vi "Decompose VI (Path).vi"(8 "Error in":errorcluster caption="Error in (no error)", 11 "VI path":path) -> (0 "Error out":errorcluster, 1 "Block Diagram XML":string, 2 "Front Panel XML":string, 3 "VI path out":path, 4 "Other resources":T1)   [LabVIEW 2023]
uses:
  CTLs/Resource Array.ctl
  CTLs/Resource.ctl
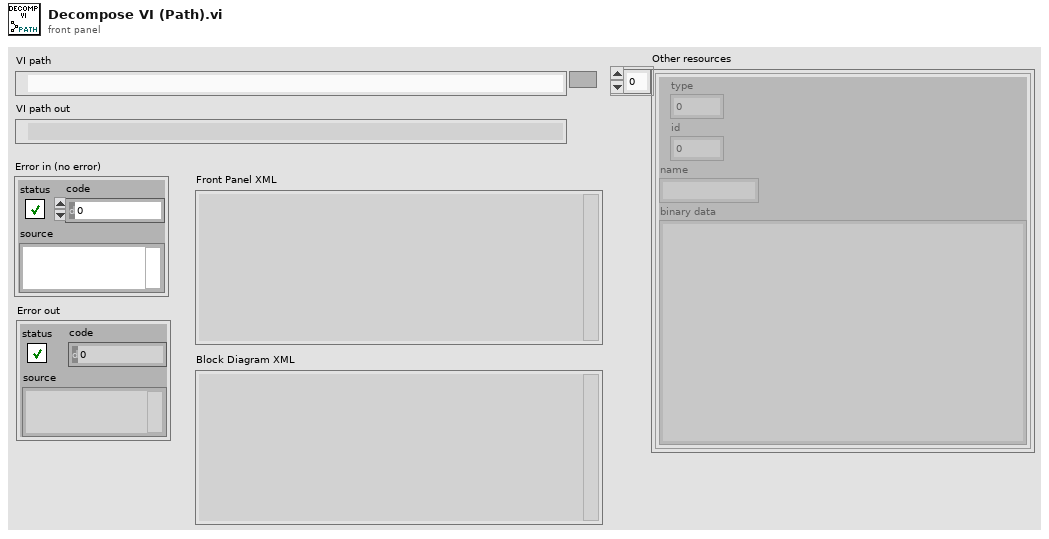
[diagram p1: front panel]
types:
  T1 = typedef "Resource Array.ctl" = T2[]
  T2 = typedef "Resource.ctl" = cluster{"type":u32, "id":i32, "name":string, "binary data":string}
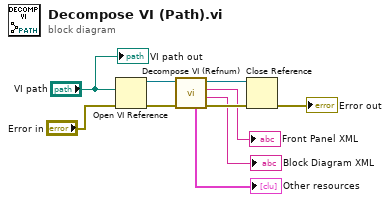
[diagram p0: block diagram]
diagram:
  n1 = Open VI Reference(vi path="VI path", error in (no error)="Error in") -> (vi reference=w10:refnum<vi>, error out=w9:errorcluster)  [unwired: 4 in]
  n2 = call "Decompose VI (Refnum).vi"("Error in"=w9, "VI Refnum"=w10) -> ("Error out"=w6:errorcluster, "Block Diagram XML"=→"Block Diagram XML":string, "Front Panel XML"=→"Front Panel XML":string, "VI Refnum Out"=w7:refnum<vi>, "Other resources"=→"Other resources":T1)  [unwired: 5 in]
  n3 = Close Reference(reference=w7, error in (no error)=w6) -> (error out=→"Error out":errorcluster)
  "VI path out" <- "VI path"
